vi "datos al Motor uni bi.vi"(8 "error in (no error)":errorcluster, 10 "Montura":T6(ring), 11 "Datos de Nueva Adquisición":T1 {"Datos Osciloscopio"."Número Promedio" min=2 max=20; "Datos a Guardar In"."Posición Actual" format="%#_10f"; "Datos a Guardar In"."Posición Cero" format="%#_10f"; "Datos Bipolar/Unipolar"."Numero de lecturas" max=910098 step=1}) -> (0 "error out":errorcluster, 3 "Datos de Nueva Adquisición OUT":T1 {"Datos Osciloscopio"."Número Promedio" min=2 max=20; "Datos a Guardar In"."Posición Actual" format="%#_10f"; "Datos a Guardar In"."Posición Cero" format="%#_10f"; "Datos Bipolar/Unipolar"."Numero de lecturas" max=910098 step=1})   [LabVIEW 2016]
uses:
  Type Definitions/Datos Zaber.ctl
  Type Definitions/parametros motores.ctl
  Type Definitions/Datos a Guardar.ctl
  Type Definitions/datos osciloscopio.ctl
  Type Definitions/Asistente de adquisicion Cluster.ctl
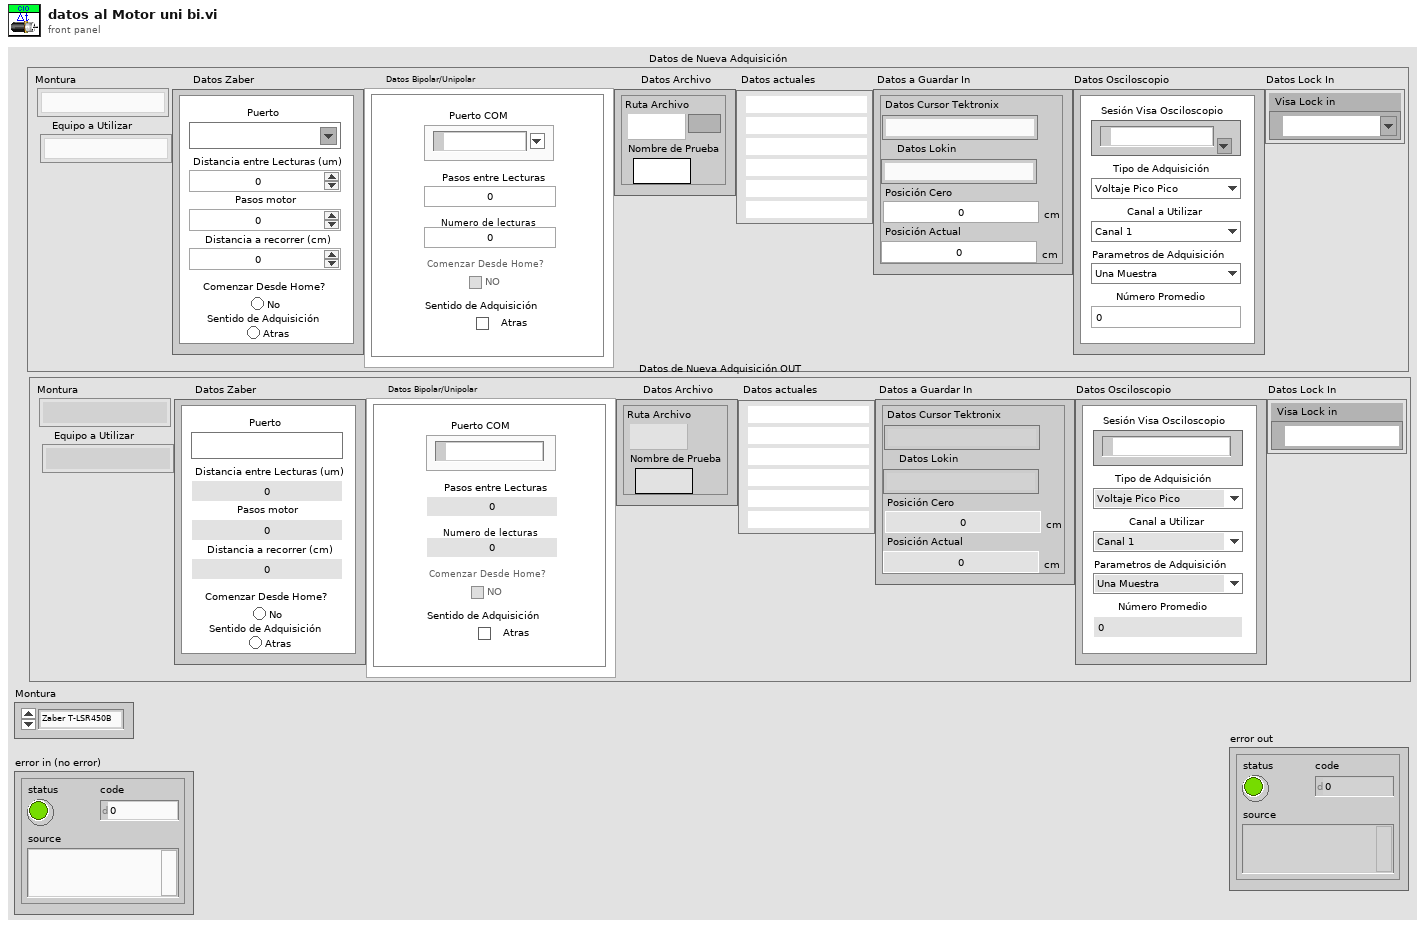
[diagram p1: front panel]
types:
  T1 = typedef "Asistente de adquisicion Cluster.ctl" = cluster{"Montura":enum16{"Zaber T-LSR450B", "Motor Bipolar", "Motor Unipolar"}, "Equipo a Utilizar":enum16{"SR830 Lock In", "TDS 2012B Osciloscope"}, "Datos Zaber":T2, "Datos Bipolar/Unipolar":T3, "Datos Archivo":cluster{"Ruta Archivo":path, "Nombre de Prueba":string}, "Datos actuales":cluster{"Montura":string, "Equipo":string, "Posición Actual":string, "Distancia Total a recorrer":string, "distancia Entre lecturas":string, "Pasos entre lecturas":string}, "Datos a Guardar In":T4, "Datos Osciloscopio":T5, "Datos Lock In":cluster{"Visa Lock in":refnum<visa-resource-name>}}
  T2 = typedef "Datos Zaber.ctl" = cluster{"Sentido de Adquisición":bool, "Comenzar Desde Home?":bool, "Distancia a recorrer (cm)":u32, "Pasos motor":i32, "Distancia entre Lecturas (um)":dbl, "Puerto":refnum<visa-resource-name>}
  T3 = typedef "parametros motores.ctl" = cluster{"Puerto COM":refnum<visa-resource-name>, "Pasos entre Lecturas":u16, "Numero de lecturas":u32, "Comenzar Desde Home?":bool, "Sentido de Adquisición":bool}
  T4 = typedef "Datos a Guardar.ctl" = cluster{"Datos Cursor Tektronix":string, "Datos Lokin":string, "Posición Cero":dbl[unit], "Posición Actual":dbl[unit]}
  T5 = typedef "datos osciloscopio.ctl" = cluster{"Sesión Visa Osciloscopio":refnum<visa-resource-name>, "Tipo de Adquisición":enum16{"Voltaje Pico Pico", "Voltaje RMS", "Cursor Tiempo"}, "Canal a Utilizar":enum16{"Canal 1", "Canal 2", "Canal 1 y 2"}, "Parametros de Adquisición":enum16{"Una Muestra", "Promedio"}, "Número Promedio":i32}
  T6 = enum16{"Zaber T-LSR450B", "Motor Bipolar", "Motor Unipolar"}
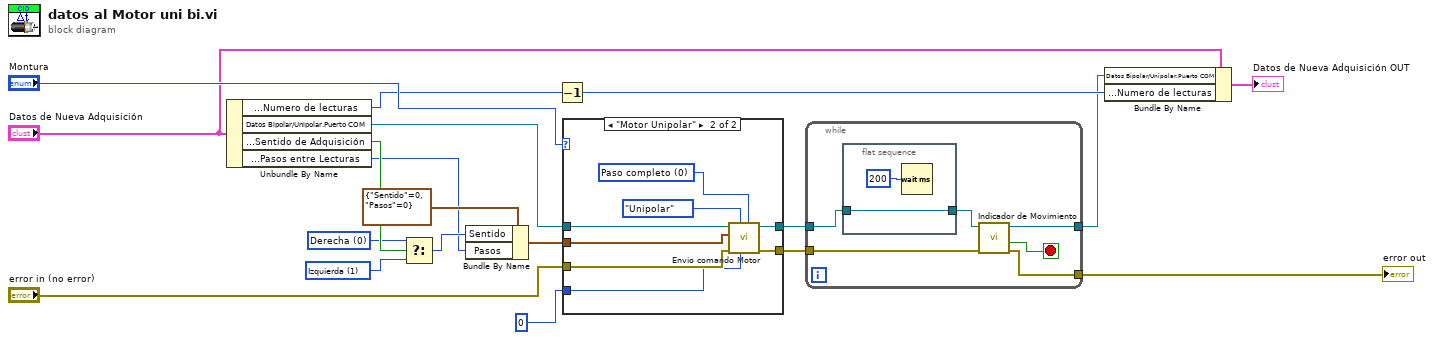
[diagram p0: block diagram]
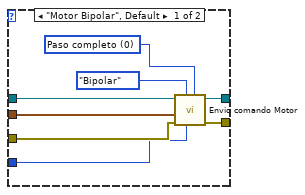
[diagram p2: hidden frame]
diagram:
  w12 = u8 1 items=["Derecha ", "Izquierda"] ("Sentido")
  w13 = u8 0 items=["Derecha ", "Izquierda"] ("Sentido")
  n1 = Unbundle By Name("Datos de Nueva Adquisición") -> ("Datos Bipolar/Unipolar.Numero de lecturas"=w8:u32, "Datos Bipolar/Unipolar.Puerto COM"=w18:refnum<visa-resource-name>, "Datos Bipolar/Unipolar.Sentido de Adquisición"=w14:bool, "Datos Bipolar/Unipolar.Pasos entre Lecturas"=w1:u16)
  n2 = Select(t=w13, s=w14, f=w12) -> (s? t:f=w15:u8)
  n3 = Bundle By Name(cluster=cluster{"Sentido":u8, "Pasos":u16} {"Sentido"=0, "Pasos"=0} ("Unipolar"), "Sentido"=w15, "Pasos"=w1) -> (w11:cluster{"Sentido":u8, "Pasos":u16})
  n4 = Decrement(x=w8) -> (x-1=w7:u32)
  n5 = case shown="\"Motor Unipolar\"" "Montura" {
    tunnel: "error in (no error)" -> [w27 w35]
    tunnel: [w26 w34] -> w4
    tunnel: w18 -> [w25 w33]
    tunnel: w11 -> [w22 w30]
    tunnel: [w21 w29] -> w6
    tunnel: u8 0 ("Velocidad(15)") -> [w20 w28]
    frame "Motor Bipolar", Default {
      w23 = u8 0 items=["Paso completo", "Medio paso"] ("Tipo de paso")
      n6 = call <instrlib>:"Envio comando Motor.vi"("Tipo de paso"=w23, "Velocidad(15)"=w20, "Seleccion Motor."=enum8{"Unipolar", "Bipolar", "Unip y Bipo"}."Bipolar", "error in (no error)"=w27, "Bipolar"=w22, "VISA resource name"=w25) -> ("error out"=w26:errorcluster, "VISA resource name out"=w21:refnum<visa-resource-name>)  [unwired: 4 in]
    }
    frame "Motor Unipolar" {
      w31 = u8 0 items=["Paso completo", "Medio paso"] ("Tipo de paso")
      n7 = call <instrlib>:"Envio comando Motor.vi"("Tipo de paso"=w31, "Velocidad(15)"=w28, "Seleccion Motor."=enum8{"Unipolar", "Bipolar", "Unip y Bipo"}."Unipolar", "error in (no error)"=w35, "Unipolar"=w30, "VISA resource name"=w33) -> ("error out"=w34:errorcluster, "VISA resource name out"=w29:refnum<visa-resource-name>)  [unwired: 4 in]
    }
  }
  n8 = while {
    tunnel: w6 -> [w38]
    tunnel: [w41] -> w5
    tunnel: w4 -> [w40]
    tunnel: [w39] -> w3
    stop <- w36 stop-if-true
    n9 = flat-sequence {
      tunnel: w38 -> [w42]
      tunnel: [w42] -> w37
      frame #0 {
        n10 = Wait (ms)(milliseconds to wait=u32 200) -> ()  [unwired: 1 out]
      }
    }
    n11 = call <instrlib>:"Indicador de Movimiento.vi"("error in (no error)"=w40, "VISA resource name"=w37) -> ("error out"=w39:errorcluster, "Paro"=w36:bool, "VISA resource name 1"=w41:refnum<visa-resource-name>)  [unwired: 6 in, 1 out]
  }
  "error out" <- w3
  n12 = Bundle By Name(cluster="Datos de Nueva Adquisición", "Datos Bipolar/Unipolar.Puerto COM"=w5, "Datos Bipolar/Unipolar.Numero de lecturas"=w7) -> (→"Datos de Nueva Adquisición OUT":T1)
